vi "run_grab_video.vi"(11 "Input":bool) -> ()   [LabVIEW 2015]
panel:
  in  "Path":path=path "D:/PROIECT DRONA/Control_drona_19.11.2016/grab_video_in_parallel.vi"
  in  "Started?":bool
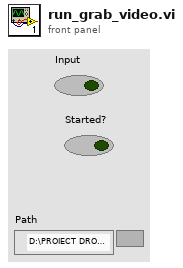
[diagram p1: front panel]
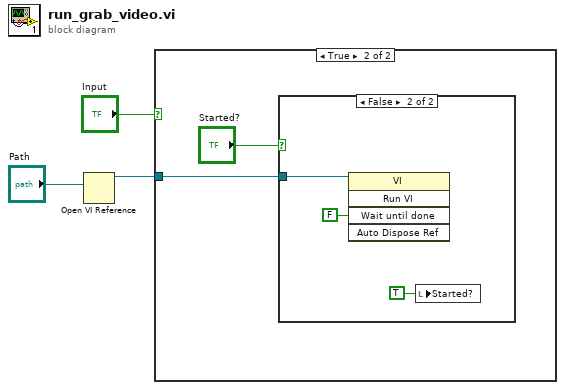
[diagram p0: block diagram]
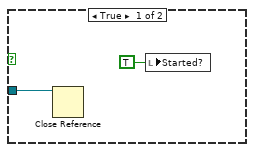
[diagram p3: hidden frame]
diagram:
  n1 = Open VI Reference(vi path="Path") -> (vi reference=w2:refnum<vi>)  [unwired: 5 in, 1 out]
  n2 = case shown="True" "Input" {
    tunnel: w2 -> [_ w4]
    frame False {
    }
    frame True {
      n3 = case shown="False" "Started?" {
        tunnel: w4 -> [w7 w10]
        frame True {
          n4 = Close Reference(reference=w7) -> ()  [unwired: 1 in, 1 out]
          n5 = local write "Started?"(TRUE) -> ()
        }
        frame False {
          n6 = invoke class="VI" method="Run VI"(reference=w10, "Wait until done"=FALSE ("Wait Until Done")) -> ()  [unwired: 3 in, 5 out]
          n7 = local write "Started?"(TRUE) -> ()
        }
      }
    }
  }
